vi "Configure Timebase.vi"(5 "Config.Model":T1, 7 "Record Length (10: 10k points)":u32(ring)=10 items=["1000 points"=1, "10k points"=10, "100k points"=100, "1M points"=1000, "5M points"=5000, "10M points"=10000], 8 "error in (no error)":errorcluster, 9 "Position (10 %)":dbl=10.0, 10 "Timebase (0.0005 s)":dbl=0.0005, 11 "VISA resource name":refnum<visa-resource-name>) -> (0 "error out":errorcluster, 3 "VISA resource name out":refnum<visa-resource-name>)   [LabVIEW 2017, in "Scope.lvlib"]
doc: "Configures the timebase and horizontal properties of the oscilloscope."
uses:
  Scope.lvlib
  Controls/Models.ctl
  Third Party Drivers/Tektronix DPO MSO 2000 4000 Series/Tektronix DPO MSO 2000 4000 Series.lvlib
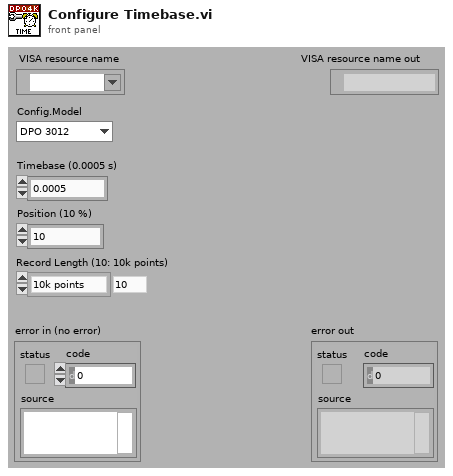
[diagram p1: front panel]
types:
  T1 = typedef "Scope.lvlib/Models.ctl" = enum16{"DPO 3012", "DPO 2012B", "TDS 3012C"}
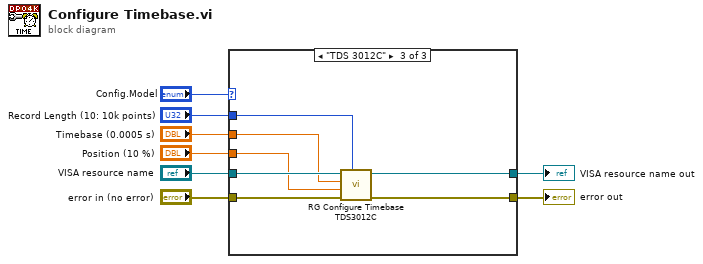
[diagram p0: block diagram]
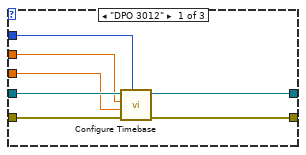
[diagram p2: hidden frame]
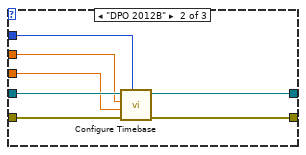
[diagram p3: hidden frame]
diagram:
  n1 = case shown="\"TDS 3012C\"" "Config.Model" {
    tunnel: "error in (no error)" -> [w15 w22 w29]
    tunnel: [w14 w21 w28] -> w6
    tunnel: "VISA resource name" -> [w13 w20 w27]
    tunnel: [w12 w19 w26] -> w4
    tunnel: "Record Length (10: 10k points)" -> [w11 w18 w23]
    tunnel: "Timebase (0.0005 s)" -> [w10 w17 w25]
    tunnel: "Position (10 %)" -> [w9 w16 w24]
    frame "DPO 3012" {
      n2 = call "Configure Timebase.vi"("Record Length (10: 10k points)"=w11, "error in (no error)"=w15, "Position (10 %)"=w9, "Timebase (0.0005 s)"=w10, "VISA resource name"=w13) -> ("error out"=w14:errorcluster, "VISA resource name out"=w12:refnum<visa-resource-name>)  [unwired: 5 in]
    }
    frame "DPO 2012B" {
      n3 = call "Configure Timebase.vi"("Record Length (10: 10k points)"=w18, "error in (no error)"=w22, "Position (10 %)"=w16, "Timebase (0.0005 s)"=w17, "VISA resource name"=w20) -> ("error out"=w21:errorcluster, "VISA resource name out"=w19:refnum<visa-resource-name>)  [unwired: 5 in]
    }
    frame "TDS 3012C" {
      n4 = call "RG Configure Timebase TDS3012C.vi"("Record Length (10: 10k points)"=w23, "error in (no error)"=w29, "Position (10 %)"=w24, "Timebase (0.0005 s)"=w25, "VISA resource name"=w27) -> ("error out"=w28:errorcluster, "VISA resource name out"=w26:refnum<visa-resource-name>)  [unwired: 5 in]
    }
  }
  "error out" <- w6
  "VISA resource name out" <- w4
